vi "球体表面积.vi"(11 "Radious":dbl) -> (3 "Area":dbl=nan)   [LabVIEW 2012]
doc: "功能：\n计算球体表面积。\n\n公式：\ns=4*Pi*r^2\n\ncsxcs_366创建"
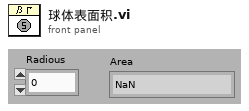
[diagram p1: front panel]
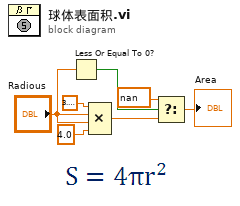
[diagram p0: block diagram]
diagram:
  n1 = Less Or Equal To 0?(x="Radious") -> (x <= 0?=w7:bool)
  n2 = Compound Arithmetic op=MULTIPLY(3.141592653589793, "Radious", "Radious", 4.0 ("值")) -> (w3:dbl)
  n3 = Select(t=nan, s=w7, f=w3) -> (s? t:f=→"Area":dbl)
